vi "GEA2 Board ID to Board Index.vi"(0 "Board ID":string, 11 "Error In":errorcluster) -> (4 "Board Found?":bool, 6 "Report Text":string="Board not found.", 8 "Board Index":i32=-1, 10 "Boards Found":string[](array[string]), 15 "Error Out":errorcluster)   [LabVIEW 2014, in "GEA2_Toolkit.lvlib"]
doc: "This VI should be placed before the GEA2 Initialize VI. This VI will output the corresponding GEA2 bus index for a given NewFI board ID input."
uses:
  library/GEA2_Toolkit.lvlib
  C:/Automation/DLLs/Appliance .NET/GeaCommunication.dll
  Automation/DLLs/Appliance .NET/GeaCommunication.dll
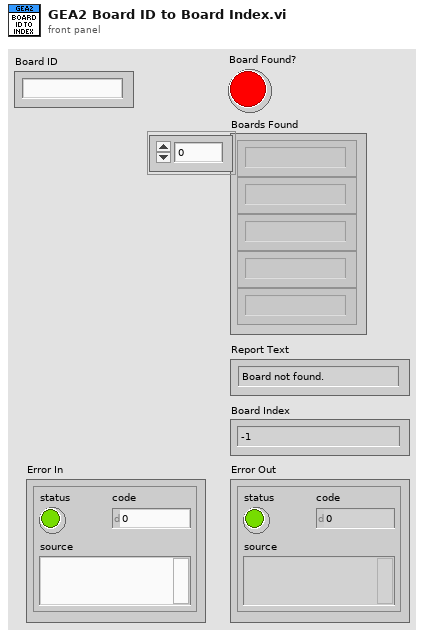
[diagram p1: front panel]
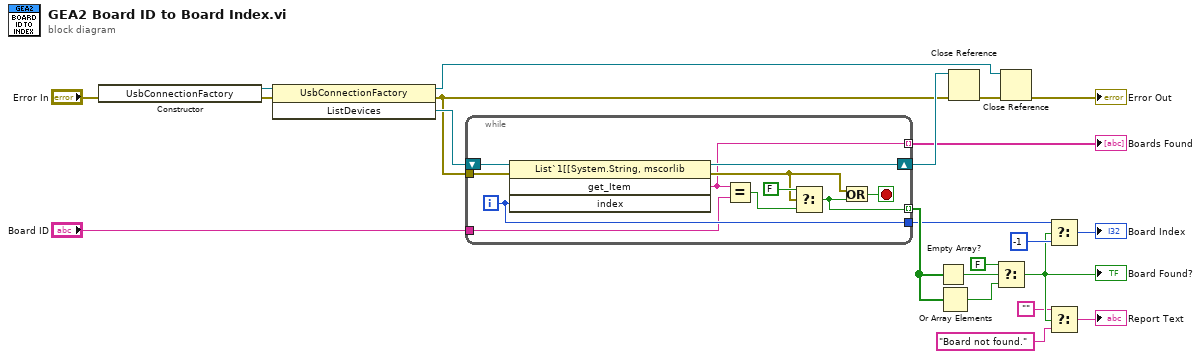
[diagram p0: block diagram]
diagram:
  n1 = constructor class="UsbConnectionFactory"(error in="Error In") -> (reference out=w22:refnum<k24>, error out=w21:errorcluster)  [unwired: 2 in, 1 out]
  n2 = invoke class="UsbConnectionFactory" method="ListDevices"(reference=w22, error in=w21) -> (reference out=w15:refnum<k24>, error out=w14:errorcluster, "ListDevices"=w20:refnum<k24>)  [unwired: 1 in]
  n3 = while {
    shift-right: [w32] -> w16
    shift-left: w20 -> [w33]
    tunnel: "Board ID" -> [w30]
    tunnel: [w31] -> w7
    tunnel: [w25] -> w12 mode=indexing
    tunnel: w14 -> [w29]
    tunnel: [w23] -> w1 mode=indexing
    i -> [w31]
    stop <- w24 stop-if-true
    n4 = invoke class="List`1[[System.String, mscorlib" method="get_Item"(reference=w33, error in=w29, "index"=w31) -> (reference out=w32:refnum<k24>, error out=w26:errorcluster, "get_Item"=w23:string)  [unwired: 1 in, 1 out]
    n5 = Equal?(x=w23, y=w30) -> (x = y?=w28:bool)
    n6 = Select(t=FALSE, s=w26, f=w28) -> (s? t:f=w25:bool)
    n7 = Or(x=w26, y=w25) -> (x .or. y?=w24:bool)
  }
  "Boards Found" <- w1
  n8 = Empty Array?(array=w12) -> (empty?=w11:bool)
  n9 = Or Array Elements(Boolean array=w12) -> (logical OR=w10:bool)
  n10 = Close Reference(reference=w16, error in (no error)=w14) -> (error out=w18:errorcluster)
  n11 = Select(t=FALSE, s=w11, f=w10) -> (s? t:f=w6:bool)
  "Board Found?" <- w6
  n12 = Close Reference(reference=w15, error in (no error)=w18) -> (error out=→"Error Out":errorcluster)
  n13 = Select(t=w7, s=w6, f=-1 ("t")) -> (s? t:f=→"Board Index":i32)
  n14 = Select(t="", s=w6, f="Board not found.") -> (s? t:f=→"Report Text":string)
